vi "PQsetdbLogin.vi"(4 "pwd":string, 5 "login":string, 6 "dbName":string, 7 "pgtty":string, 8 "error in (no error)":errorcluster, 9 "pgoptions":string, 10 "pgport":string, 11 "pghost":string) -> (0 "error out":errorcluster, 3 "conn":u32)   [LabVIEW 2019, in "libpqlv.lvlib"]
doc: "Makes a new connection to the database server.\nThis is the predecessor of PQconnectdb with a fixed set of parameters. It has the same functionality except that the missing parameters will always take on default values. Write NULL or an empty string for any one of the fixed parameters that is to be defaulted."
uses:
  libpqlv.lvlib
  libpq.dll
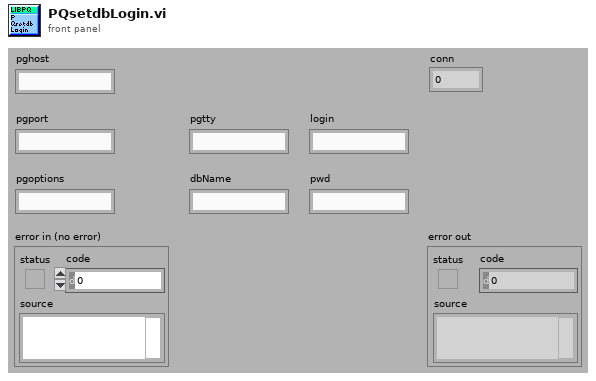
[diagram p1: front panel]
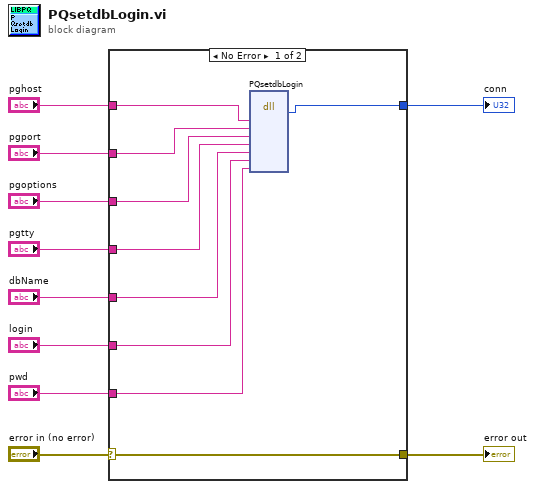
[diagram p0: block diagram]
diagram:
  n1 = case shown="No Error" "error in (no error)" {
    selector: "error in (no error)" -> [w19 w20]
    tunnel: [w19 w20] -> w9
    tunnel: [w18 _] -> w8
    tunnel: "pghost" -> [w17 _]
    tunnel: "pgport" -> [w16 _]
    tunnel: "pgoptions" -> [w15 _]
    tunnel: "pgtty" -> [w14 _]
    tunnel: "dbName" -> [w13 _]
    tunnel: "login" -> [w12 _]
    tunnel: "pwd" -> [w11 _]
    frame No Error {
      n2 = dll-call lib="libpq.*" fn="PQsetdbLogin"("pghost"=w17, "pgport"=w16, "pgoptions"=w15, "pgtty"=w14, "dbName"=w13, "login"=w12, "pwd"=w11) -> ("return type"=w18:u32)  [unwired: 10 in, 2 out]
    }
    frame Error {
    }
  }
  "conn" <- w8
  "error out" <- w9
